vi "Convert String Array to Cluster.vi"(10 "# of Channels":i32, 11 "IO Names":string[](array[string])) -> (3 "Variant":variant)   [LabVIEW 2015, in "Module.lvclass"]
uses:
  Module.lvclass
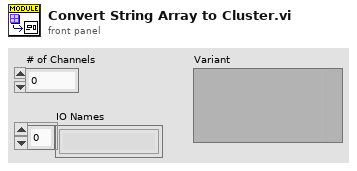
[diagram p1: front panel]
types:
  T1 = cluster{"IO Names[0]":string, "IO Names[1]":string, "IO Names[2]":string, "IO Names[3]":string}
  T2 = cluster{"IO Names[0]":string, "IO Names[1]":string, "IO Names[2]":string, "IO Names[3]":string, "IO Names[4]":string, "IO Names[5]":string, "IO Names[6]":string, "IO Names[7]":string}
  T3 = cluster{"IO Names[0]":string, "IO Names[1]":string, "IO Names[2]":string, "IO Names[3]":string, "IO Names[4]":string, "IO Names[5]":string, "IO Names[6]":string, "IO Names[7]":string, "IO Names[8]":string, "IO Names[9]":string, "IO Names[10]":string, "IO Names[11]":string, "IO Names[12]":string, "IO Names[13]":string, "IO Names[14]":string, "IO Names[15]":string}
  T4 = cluster{"IO Names[0]":string, "IO Names[1]":string, "IO Names[2]":string, "IO Names[3]":string, "IO Names[4]":string, "IO Names[5]":string, "IO Names[6]":string, "IO Names[7]":string, "IO Names[8]":string, "IO Names[9]":string, "IO Names[10]":string, "IO Names[11]":string, "IO Names[12]":string, "IO Names[13]":string, "IO Names[14]":string, "IO Names[15]":string, "IO Names[16]":string, "IO Names[17]":string, "IO Names[18]":string, "IO Names[19]":string, "IO Names[20]":string, "IO Names[21]":string, "IO Names[22]":string, "IO Names[23]":string, "IO Names[24]":string, "IO Names[25]":string, "IO Names[26]":string, "IO Names[27]":string, "IO Names[28]":string, "IO Names[29]":string, "IO Names[30]":string, "IO Names[31]":string}
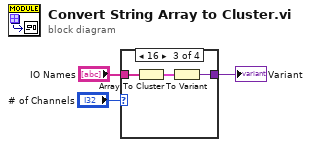
[diagram p0: block diagram]
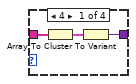
[diagram p2: hidden frame]
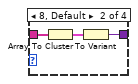
[diagram p3: hidden frame]
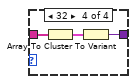
[diagram p4: hidden frame]
diagram:
  n1 = case shown="16" "# of Channels" {
    tunnel: "IO Names" -> [w6 w9 w12 w15]
    tunnel: [w5 w8 w11 w14] -> w2
    frame 4 {
      n2 = Array To Cluster(array=w6) -> (cluster=w4:T1)
      n3 = To Variant(anything=w4) -> (Variant=w5:variant)
    }
    frame 8, Default {
      n4 = Array To Cluster(array=w9) -> (cluster=w7:T2)
      n5 = To Variant(anything=w7) -> (Variant=w8:variant)
    }
    frame 16 {
      n6 = Array To Cluster(array=w12) -> (cluster=w10:T3)
      n7 = To Variant(anything=w10) -> (Variant=w11:variant)
    }
    frame 32 {
      n8 = Array To Cluster(array=w15) -> (cluster=w13:T4)
      n9 = To Variant(anything=w13) -> (Variant=w14:variant)
    }
  }
  "Variant" <- w2
